vi "Reverse2DArray.vi"(1 "2D Array":string[][](array[string])) -> (0 "Reversed 2D Array":string[][](array[string]))   [LabVIEW 2013]
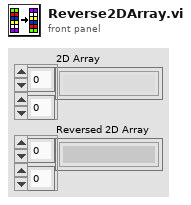
[diagram p1: front panel]
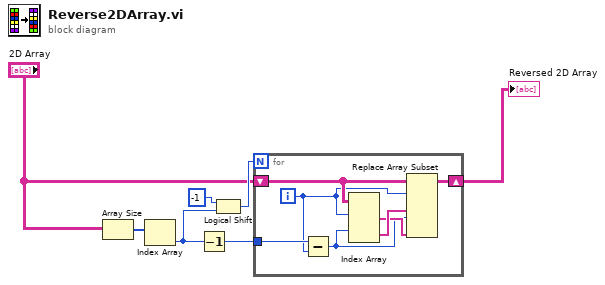
[diagram p0: block diagram]
diagram:
  n1 = Array Size(array="2D Array") -> (size(s)=w7:i32[])
  n2 = Index Array(array=w7) -> (element=w5:i32)  [unwired: 1 in]
  n3 = Decrement(x=w5) -> (x-1=w3:i32)
  n4 = Logical Shift(y=i8 -1, x=w5) -> (x << y=w6:i32)
  n5 = for {
    N: w6 -> [_]
    shift-right: [w14] -> w1
    shift-left: "2D Array" -> [w13]
    tunnel: w3 -> [w10]
    i -> [w9]
    n6 = Subtract(x=w10, y=w9) -> (x-y=w8:i32)
    n7 = Index Array(array=w13, index (row) #1=w9, index (row) #2=w8) -> (element #1=w11:string[], element #2=w12:string[])  [unwired: 2 in]
    n8 = Replace Array Subset(array=w13, new element #1=w12, index (row) #1=w9, new element #2=w11, index (row) #2=w8) -> (w14:string[][])  [unwired: 2 in]
  }
  "Reversed 2D Array" <- w1
